vi "Get Data.vi"(8 "error in":errorcluster, 11 "AlicatPData in":refnum<class "AlicatPData.lvclass">) -> (0 "error out":errorcluster, 2 "DataOut":cluster{"P":dbl, "dP":dbl, "Q":dbl}, 3 "AlicatPData out":refnum<class "AlicatPData.lvclass">)   [LabVIEW 2014, in "Alicat.lvlib" / "AlicatPData.lvclass"]
uses:
  AlicatPData.lvclass
  AlicatPData.lvclass/AlicatPData.ctl
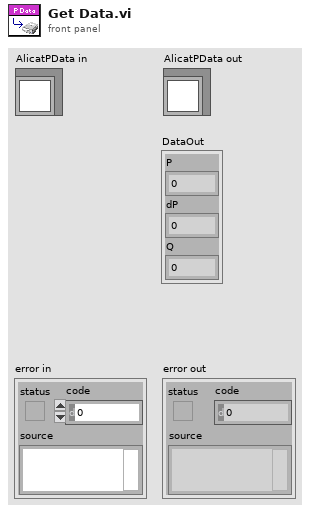
[diagram p1: front panel]
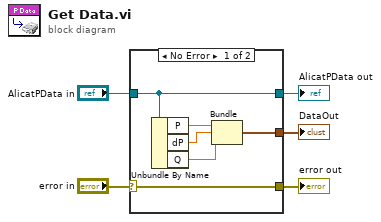
[diagram p0: block diagram]
diagram:
  n1 = case shown="No Error" "error in" {
    selector: "error in" -> [w11 w13]
    tunnel: [w11 w13] -> w4
    tunnel: [w10 w12] -> w2
    tunnel: "AlicatPData in" -> [w10 w12]
    tunnel: [w6 _] -> w1
    frame No Error {
      n2 = Unbundle By Name(w10) -> ("P"=w9:dbl, "dP"=w8:dbl, "Q"=w7:dbl)
      n3 = Bundle("P"=w9, "dP"=w8, "Q"=w7) -> (w6:cluster{"P":dbl, "dP":dbl, "Q":dbl})  [unwired: 1 in]
    }
    frame Error {
    }
  }
  "error out" <- w4
  "AlicatPData out" <- w2
  "DataOut" <- w1
